vi "SendSetDigitalPWMCommand.vi"(6 "Pin [0 - 11]":u8=1 max=11, 7 "Value [0 - 255]":u8=1, 8 "entrée d'erreur (pas d'erreur)":errorcluster, 9 "Port Distant":u16, 10 "Numérique":u32, 11 "Connexion réseau UDP en entrée":refnum<k16>) -> ()   [LabVIEW 2021]
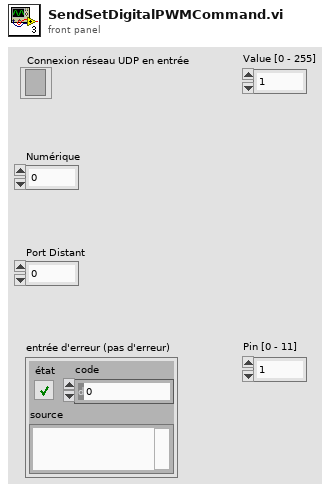
[diagram p1: front panel]
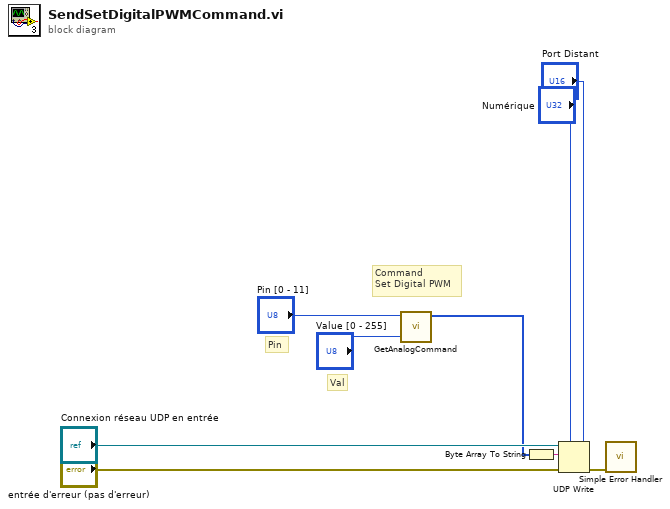
[diagram p0: block diagram]
diagram:
  # "Command \nSet Digital PWM"
  # "Val"
  # "Pin"
  n1 = call "GetAnalogCommand.vi"("Numérique"="Value [0 - 255]", "Numérique 2"="Pin [0 - 11]") -> ("Tableau"=w4:u8[])  [unwired: 9 in]
  n2 = Byte Array To String(unsigned byte array=w4) -> (string=w1:string)
  n3 = UDP Write(address="Numérique", port or service name="Port Distant", connection ID="Connexion réseau UDP en entrée", data in=w1, 8:"entrée d'erreur (pas d'erreur)") -> (error out=w2:errorcluster)  [unwired: 1 in, 1 out]
  n4 = call <vilib>:"Simple Error Handler.vi"("error in (no error)"=w2) -> ()  [unwired: 4 in, 5 out]
